vi "LED different Color chnage.vi"() -> ()   [LabVIEW 2015]
panel:
  in  "Tab Control 2":enum32{"Page 1", "Page 2"}(tab)
  in  "Cluster":T1
  in  "Color Box":u32(colorbox)
  in  "Color Box 2":u32(colorbox)
  in  "Color Box 3":u32(colorbox)
  in  "stop 2":bool
  in  "Enum":enum16{"Blue", "Black", "Green", "Red"}(ring)
  out "Cluster 2":cluster{"Boolean":bool}
  in  "stop":bool
  # "LED different Color chnage"
  # "Pardeep Kumar"
  # "Pardeep Kumar"
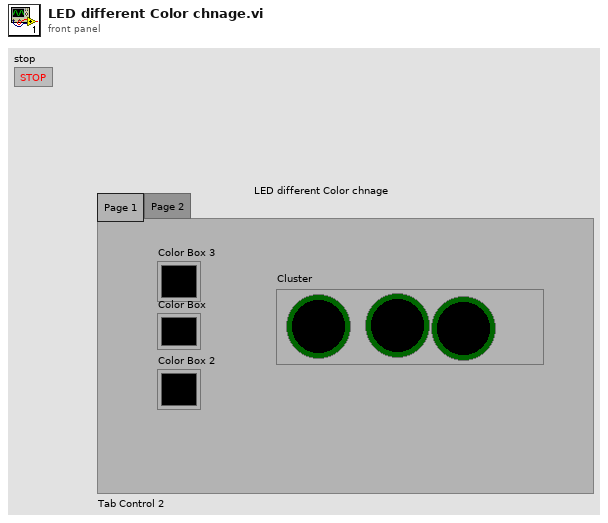
[diagram p1: front panel]
types:
  T1 = cluster{"Boolean 2":bool, "Boolean 3":bool, "Boolean":bool}
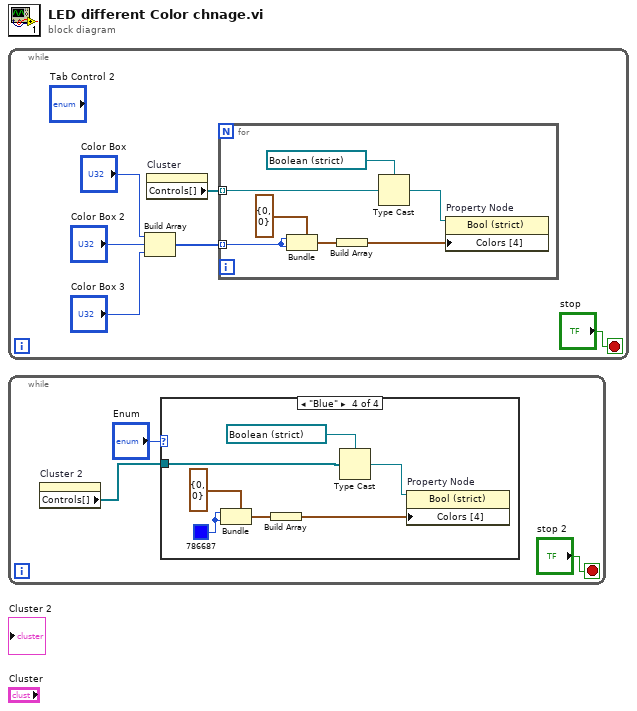
[diagram p0: block diagram]
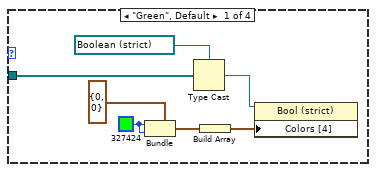
[diagram p2: hidden frame]
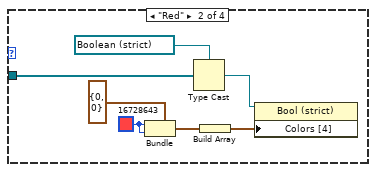
[diagram p3: hidden frame]
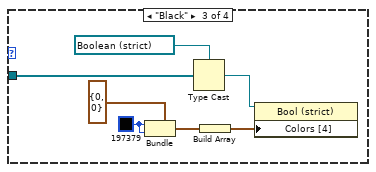
[diagram p4: hidden frame]
diagram:
  n1 = while {
    stop <- "stop" stop-if-true
    n2 = Build Array "Build Array"("Color Box", "Color Box 2", "Color Box 3") -> (w1:u32[])
    n3 = property on="Cluster" class="Clust (strict)"() -> ("Controls[]"=w2:refnum<vi>[])  [unwired: 2 in, 2 out]
    n4 = for {
      tunnel: w2 -> [w13] mode=indexing
      tunnel: w1 -> [w9] mode=indexing
      n5 = Bundle "Bundle"(cluster=cluster{u32, u32} {0, 0}, w9, w9) -> (w8:cluster{u32, u32})
      n6 = Build Array "Build Array"(w8) -> (w7:cluster{u32, u32}[])
      n7 = Type Cast(type=refnum<vi> refnum ("reference"), x=w13) -> (*(type *) &x=w11:refnum<vi>)
      n8 = property on="Property Node" class="Bool (strict)"(reference=w11, "Colors [4]"=w7) -> ()  [unwired: 1 in, 2 out]
    }
  }
  n9 = while {
    stop <- "stop 2" stop-if-true
    n10 = property on="Cluster 2" class="Clust (strict)"() -> ("Controls[]"=w15:refnum<vi>[])  [unwired: 2 in, 2 out]
    n11 = case shown="\"Blue\"" "Enum" {
      tunnel: w15 -> [w20 w26 w31 w38]
      frame "Green", Default {
        w17 = u32 327424
        n12 = Bundle(cluster=cluster{u32, u32} {0, 0}, w17, w17) -> (w23:cluster{u32, u32})
        n13 = Type Cast(type=refnum<vi> refnum ("reference"), x=w20) -> (*(type *) &x=w18:refnum<vi>)
        n14 = Build Array(w23) -> (w21:cluster{u32, u32}[])
        n15 = property on="Property Node" class="Bool (strict)"(reference=w18, "Colors [4]"=w21) -> ()  [unwired: 1 in, 2 out]
      }
      frame "Red" {
        w24 = u32 16728643
        n16 = Bundle(cluster=cluster{u32, u32} {0, 0}, w24, w24) -> (w30:cluster{u32, u32})
        n17 = Type Cast(type=refnum<vi> refnum ("reference"), x=w26) -> (*(type *) &x=w27:refnum<vi>)
        n18 = Build Array(w30) -> (w28:cluster{u32, u32}[])
        n19 = property on="Property Node" class="Bool (strict)"(reference=w27, "Colors [4]"=w28) -> ()  [unwired: 1 in, 2 out]
      }
      frame "Black" {
        w32 = u32 197379
        n20 = Bundle(cluster=cluster{u32, u32} {0, 0}, w32, w32) -> (w37:cluster{u32, u32})
        n21 = Type Cast(type=refnum<vi> refnum ("reference"), x=w31) -> (*(type *) &x=w34:refnum<vi>)
        n22 = Build Array(w37) -> (w35:cluster{u32, u32}[])
        n23 = property on="Property Node" class="Bool (strict)"(reference=w34, "Colors [4]"=w35) -> ()  [unwired: 1 in, 2 out]
      }
      frame "Blue" {
        w39 = u32 786687
        n24 = Bundle "Bundle"(cluster=cluster{u32, u32} {0, 0}, w39, w39) -> (w44:cluster{u32, u32})
        n25 = Build Array "Build Array"(w44) -> (w42:cluster{u32, u32}[])
        n26 = Type Cast(type=refnum<vi> refnum ("reference"), x=w38) -> (*(type *) &x=w41:refnum<vi>)
        n27 = property on="Property Node" class="Bool (strict)"(reference=w41, "Colors [4]"=w42) -> ()  [unwired: 1 in, 2 out]
      }
    }
  }
